vi "Configure File System.vi"(4 "Destination Path":string, 6 "Data":string, 7 "Operation (0: Set Current Working Directory)":i32(ring) items=["Set Current Working Directory", "Read File", "Rename File", "Write File", "Delete", "Create Folder"], 8 "error in (no error)":errorcluster, 9 "Path":string, 10 "Working Directory Path (\"E:/\")":string="E:/", 11 "VISA resource name":refnum<visa-resource-name>) -> (0 "error out":errorcluster, 3 "VISA resource name out":refnum<visa-resource-name>)   [LabVIEW 2009, in "Tektronix DPO MSO 2000 4000 Series.lvlib"]
doc: "Configures file sysem for an oscilloscope according to <B>Operation</B>."
uses:
  <instrlib>/Tektronix DPO MSO 2000 4000 Series/Tektronix DPO MSO 2000 4000 Series.lvlib
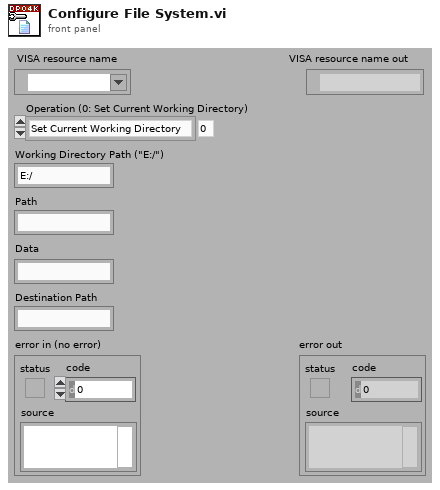
[diagram p1: front panel]
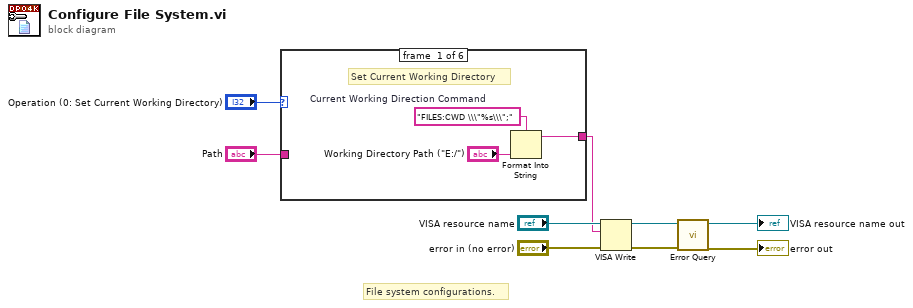
[diagram p0: block diagram]
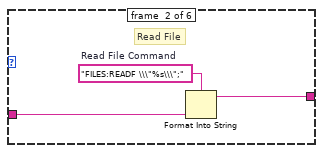
[diagram p2: hidden frame]
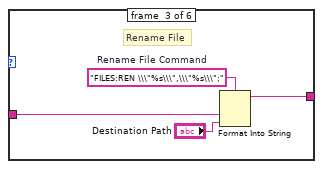
[diagram p3: hidden frame]
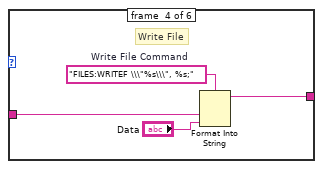
[diagram p4: hidden frame]
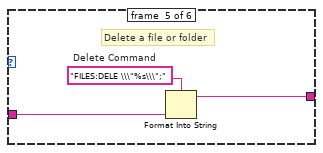
[diagram p5: hidden frame]
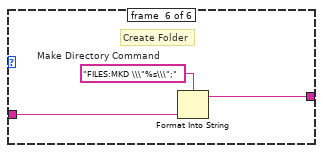
[diagram p6: hidden frame]
diagram:
  # "File system configurations."
  n1 = case shown="0, Default" "Operation (0: Set Current Working Directory)" {
    tunnel: [w11 w14 w17 w20 w24 w27] -> w2
    tunnel: "Path" -> [_ w15 w18 w22 w25 w29]
    frame #0 {
      w12 = "FILES:CWD \\\"%s\\\";"  # Current Working Direction Command
      # "Set Current Working Directory"
      n2 = Format Into String(format string=w12, "Working Directory Path (\"E:/\")") -> (resulting string=w11:string)  [unwired: 2 in, 1 out]
    }
    frame #1 {
      w13 = "FILES:READF \\\"%s\\\";"  # Read File Command
      # "Read File"
      n3 = Format Into String(format string=w13, w15) -> (resulting string=w14:string)  [unwired: 2 in, 1 out]
    }
    frame #2 {
      w19 = "FILES:REN \\\"%s\\\",\\\"%s\\\";"  # Rename File Command
      # "Rename File"
      n4 = Format Into String(format string=w19, w18, "Destination Path") -> (resulting string=w17:string)  [unwired: 2 in, 1 out]
    }
    frame #3 {
      w21 = "FILES:WRITEF \\\"%s\\\", %s;"  # Write File Command
      # "Write File"
      n5 = Format Into String(format string=w21, w22, "Data") -> (resulting string=w20:string)  [unwired: 2 in, 1 out]
    }
    frame #4 {
      w26 = "FILES:DELE \\\"%s\\\";"  # Delete Command
      # "Delete a file or folder"
      n6 = Format Into String(format string=w26, w25) -> (resulting string=w24:string)  [unwired: 2 in, 1 out]
    }
    frame #5 {
      w28 = "FILES:MKD \\\"%s\\\";"  # Make Directory Command
      # "Create Folder"
      n7 = Format Into String(format string=w28, w29) -> (resulting string=w27:string)  [unwired: 2 in, 1 out]
    }
  }
  n8 = VISA Write(VISA resource name="VISA resource name", write buffer=w2, error in (no error)="error in (no error)") -> (VISA resource name out=w7:refnum<visa-resource-name>, error out=w6:errorcluster)  [unwired: 1 out]
  n9 = call <instrlib>:"Error Query.vi"("error in (no error)"=w6, "VISA resource name"=w7) -> ("error out"=→"error out":errorcluster, "VISA resource name out"=→"VISA resource name out":refnum<visa-resource-name>)  [unwired: 6 in, 2 out]
